vi "MH_GetStartTime.vi"(8 "error in (no error)":errorcluster, 11 "devidx":i32) -> (0 "error out":errorcluster, 1 "timedw1":u32, 2 "timedw2":u32, 3 "return type":i32, 4 "timedw0":u32)   [LabVIEW 2019]
uses:
  MH_DllPath_global.vi
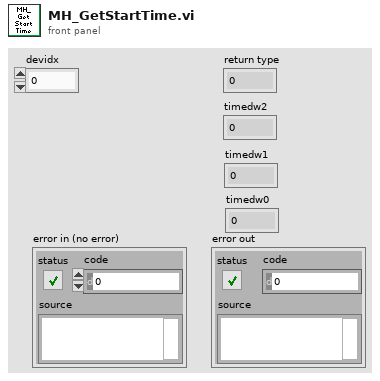
[diagram p1: front panel]
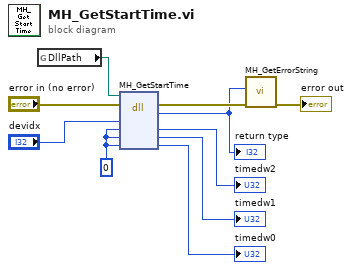
[diagram p0: block diagram]
diagram:
  w4 = u32 0 ("resolution")
  n1 = global read "MH_DllPath_global.vi" "DllPath"() -> (w9:path)
  n2 = dll-call lib="MHLib64.dll" fn="MH_GetStartTime"(path in=w9, error in="error in (no error)", "devidx"="devidx", "timedw2"=w4, "timedw1"=w4, "timedw0"=w4) -> (error out=w7:errorcluster, "return type"=w6:i32, "timedw2"=→"timedw2":u32, "timedw1"=→"timedw1":u32, "timedw0"=→"timedw0":u32)  [unwired: 2 in, 1 out]
  "return type" <- w6
  n3 = call "MH_GetErrorString.vi"("error in (no error)"=w7, "code"=w6) -> ("error out"=→"error out":errorcluster)  [unwired: 7 in, 2 out]
